vi "WLM Operation.vi"(8 "error in (no error)":errorcluster, 10 "operation (meas. mode)":T1(ring)=enum."Measurement mode") -> (0 "error out":errorcluster, 2 "return value":u32)   [LabVIEW 2023]
doc: "Sets the operation mode for the wavelength meter. Normally this should be set to \"Measurement mode.\""
uses:
  HighFinesse WS5/wlmData.dll
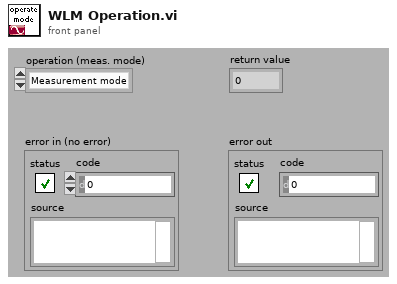
[diagram p1: front panel]
types:
  T1 = enum16{"Measurement off", "Adjustment mode", "Measurement mode"}
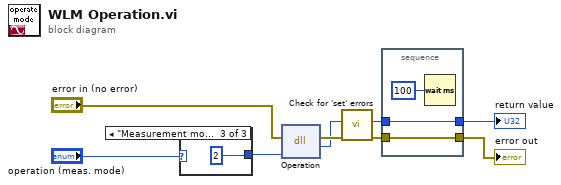
[diagram p0: block diagram]
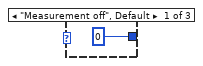
[diagram p2: hidden frame]
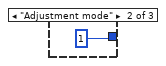
[diagram p3: hidden frame]
diagram:
  n1 = case shown="\"Measurement mode\"" "operation (meas. mode)" {
    tunnel: [u8 0 ("Res1") u8 1 ("Res1") u8 2 ("Res1")] -> w5
    frame "Measurement off", Default {
    }
    frame "Adjustment mode" {
    }
    frame "Measurement mode" {
    }
  }
  n2 = dll-call lib="C:/LabVIEW-programs/Instruments/Wavelength meter/HighFinesse WS5/wlmData.dll" fn="Operation"(error in="error in (no error)", "Op"=w5) -> (error out=w7:errorcluster, "return type"=w6:u32)  [unwired: 3 in, 1 out]
  n3 = call "Check for 'set' errors.vi"("error in (no error)"=w7, "return value"=w6) -> ("error out"=w4:errorcluster, "return value out"=w2:i32)  [unwired: 8 out]
  n4 = stacked-sequence {
    tunnel: w4 -> [w15]
    tunnel: [w15] -> w3
    tunnel: w2 -> [w14]
    tunnel: [w14] -> w1
    frame #0 {
      n5 = Wait (ms)(milliseconds to wait=u32 100) -> ()  [unwired: 1 out]
    }
  }
  "return value" <- w1
  "error out" <- w3
